vi "Alarme de temperatura - Case.vi"() -> ()   [LabVIEW 2021]
panel:
  in  "frequency (Hz)":u32
  in  "duration (msec)":u32
  in  "use system alert? (T)":bool=TRUE
  in  "Limite":dbl
  out "Média 5 últimas medidas":dbl
  in  "Temp Scale":bool
  out "Temp History":cluster{"Thermometer":dbl, dbl, "Limite":dbl}(graph)
  in  "Power":bool
  # "ON"
  # "OFF"
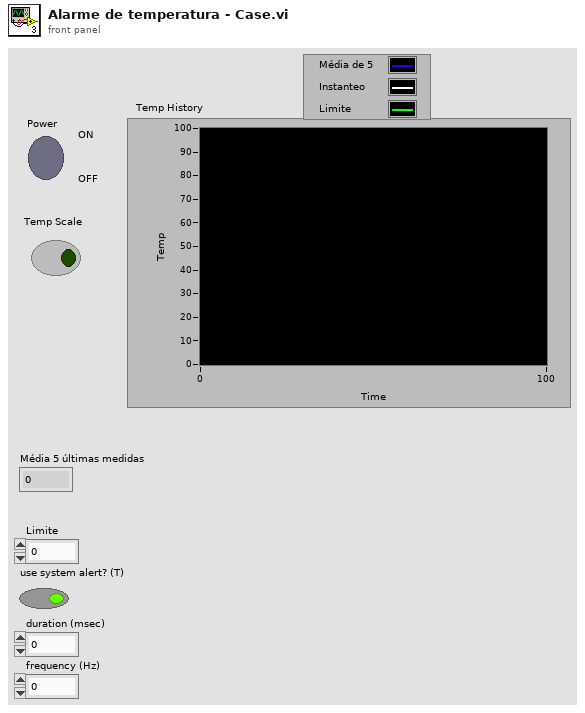
[diagram p1: front panel]
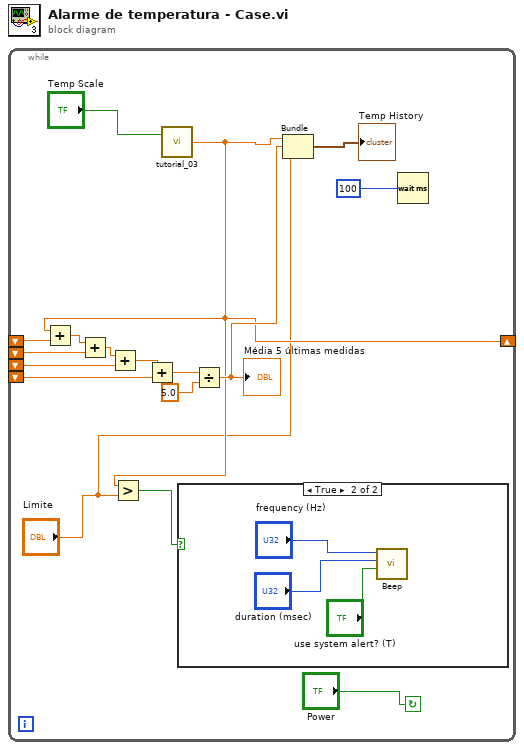
[diagram p0: block diagram]
diagram:
  n1 = while {
    shift-right: [w3] -> _
    shift-left: _ -> [w8]
    shift-left: _ -> [w14]
    shift-left: _ -> [w10]
    shift-left: _ -> [w11]
    stop <- "Power" continue-if-true
    n2 = call "tutorial_03.vi"("Temp Scale"="Temp Scale") -> ("Thermometer"=w3:dbl)  [unwired: 1 in]
    n3 = Add(x=w3, y=w14) -> (x+y=w12:dbl)
    n4 = Add(x=w12, y=w11) -> (x+y=w13:dbl)
    n5 = Add(x=w13, y=w10) -> (x+y=w9:dbl)
    n6 = Greater?(x=w3, y="Limite") -> (0:w2:bool)
    n7 = Add(x=w9, y=w8) -> (x+y=w7:dbl)
    n8 = case shown="True" w2 {
      frame False {
      }
      frame True {
        n9 = call <vilib>:"Beep.vi"("use system alert? (T)"="use system alert? (T)", "duration (msec)"="duration (msec)", "frequency (Hz)"="frequency (Hz)") -> ()  [unwired: 9 in]
      }
    }
    n10 = Divide(x=w7, y=5.0 ("x/y")) -> (x/y=w5:dbl)
    "Média 5 últimas medidas" <- w5
    n11 = Bundle("Thermometer"=w3, w5, "Limite"="Limite") -> (→"Temp History":cluster{"Thermometer":dbl, dbl, "Limite":dbl})  [unwired: 1 in]
    n12 = Wait (ms)(milliseconds to wait=u32 100 ("millisecond timer value")) -> ()  [unwired: 1 out]
  }
